vi "Close Instrument.vi"(8 "error in (no error)":errorcluster, 11 "Instrument.VoltageSource in":refnum<class "Instrument.VoltageSource.lvclass">) -> (0 "error out":errorcluster, 3 "Instrument.VoltageSource out":refnum<class "Instrument.VoltageSource.lvclass">)   [LabVIEW 2016, in "Instrument.VoltageSource.lvclass"]
uses:
  Instrument.VoltageSource.lvclass
  Instrument.VoltageSource.lvclass/Instrument.VoltageSource.ctl
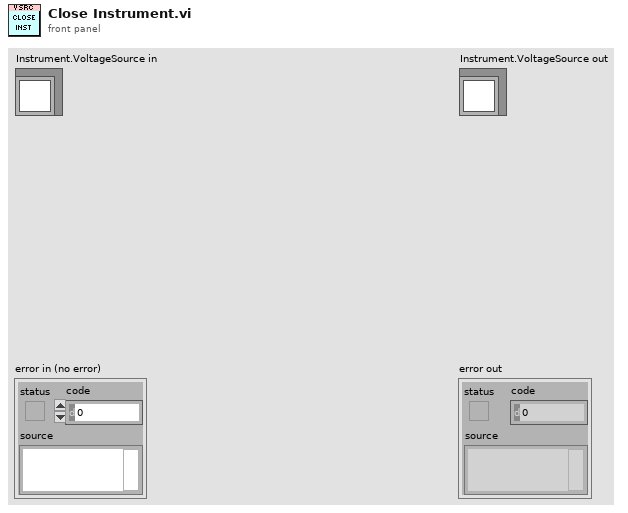
[diagram p1: front panel]
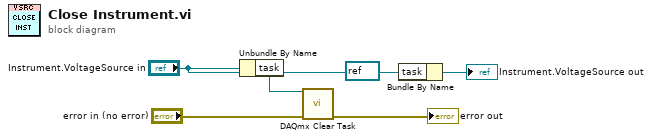
[diagram p0: block diagram]
diagram:
  n1 = Unbundle By Name("Instrument.VoltageSource in") -> ("task"=w1:refnum<k21>)
  n2 = call <vilib>:"DAQmx Clear Task.vi"("task in"=w1, "error in"="error in (no error)") -> ("error out"=→"error out":errorcluster)  [unwired: 13 in]
  n3 = Bundle By Name(cluster="Instrument.VoltageSource in", "task"=refnum<k21> refnum ("task out")) -> (→"Instrument.VoltageSource out":refnum<class "Instrument.VoltageSource.lvclass">)
